vi "ql2proto_response_type_encode.vi"(11 "response_type":T1) -> (2 "query_type_ids":u32[](array[numeric])=[1, 2, 3, 10, 11, 169, 153, 12, 13, 14, 15, 16, 78, 17, 18, 19, 20, 21, 22, 23, 24, 25, 26, 27, 28, 183, 184, 185, 29, 80, 95, 88, 89, 90, 91, 30, 70, 71, 87, 93, 31, 94, 186, 143, 32, 96, 33, 34, 35, 36, 182, 37, 38, 187, 39, 40, 41, 42, 43, 86, 44, 45, 170, 48, 49, 50, 72, 173, 82, 83, 84, 85, 51, 52, 53, 54, 55, 56, 57, 58, 59, 60, 61, 62, 174, 175, 177, 176, 179, 138, 188, 75, 76, 77, 139, 140, 156, 189, 190, 64, 65, 66, 67, 68, 69, 73, 74, 79, 97, 141, 142, 81, 92, 98, 99, 100, 101, 102, 103, 104, 105, 106, 126, 127, 128, 129, 130, 131, 132, 133, 134, 135, 136, 107, 108, 109, 110, 111, 112, 113, 114, 115, 116, 117, 118, 119, 120, 121, 122, 123, 124, 125, 137, 144, 145, 146, 147, 148, 149, 150, 151, 152, 154, 155, 157, 158, 159, 160, 161, 162, 163, 164, 165, 166, 167, 168, 171, 172, 180, 181, 191, 192, 193, 194, 195, 196], 3 "id":u32)   [LabVIEW 2017]
uses:
  ql2proto_response_type.ctl
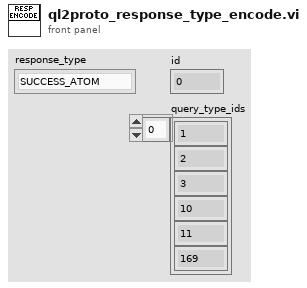
[diagram p1: front panel]
types:
  T1 = typedef "ql2proto_response_type.ctl" = enum8{"SUCCESS_ATOM", "SUCCESS_SEQUENCE", "SUCCESS_PARTIAL", "WAIT_COMPLETE", "SERVER_INFO", "CLIENT_ERROR", "COMPILE_ERROR", "RUNTIME_ERROR", "invalid"}
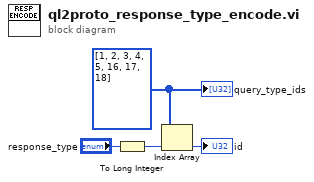
[diagram p0: block diagram]
diagram:
  w1 = u32[] [1, 2, 3, 4, 5, 16, 17, 18] ("ids")
  n1 = To Long Integer(number="response_type") -> (32bit integer=w3:i32)
  n2 = Index Array(array=w1, index=w3) -> (element=→"id":u32)
  "query_type_ids" <- w1
